vi "Assignment4_WashingMachine.vi"() -> ()   [LabVIEW 2024]
uses:
  WashingCycle.ctl
panel:
  in  "Mode":enum16{"Colourful", "Intensive", "Quick Wash"}(ring)
  in  "Start":bool
  out "Display":cluster{"Stage":string, "Time Remaining":dbl}
  in  "On/Off":bool
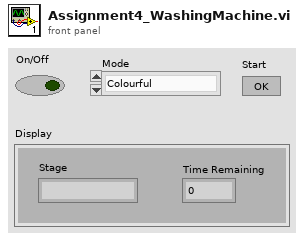
[diagram p1: front panel]
types:
  T1 = typedef "WashingCycle.ctl" = enum16{"Pre-rinse", "Main Washing", "Final Spin"}
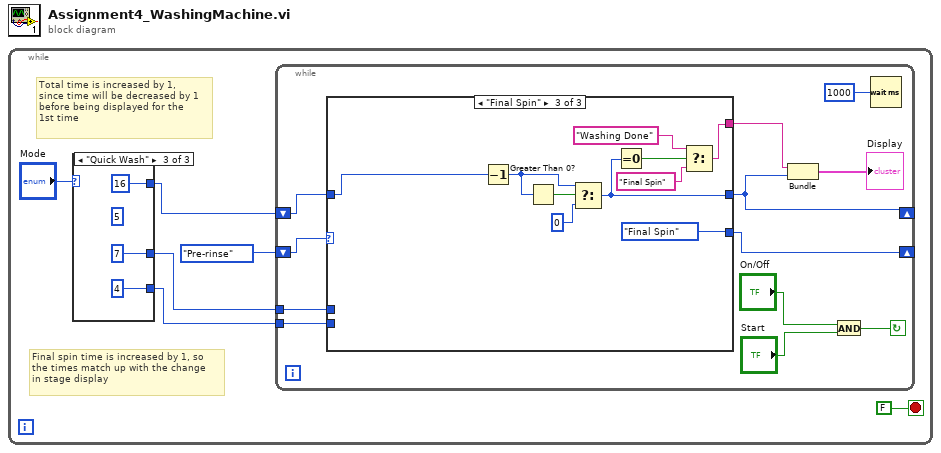
[diagram p0: block diagram]
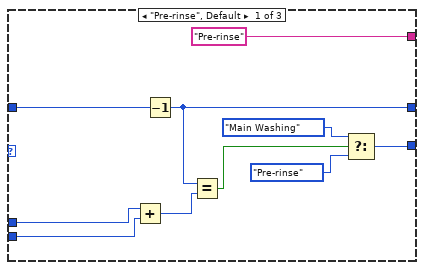
[diagram p2: hidden frame]
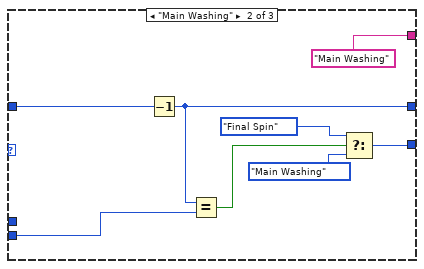
[diagram p3: hidden frame]
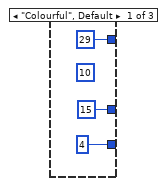
[diagram p4: hidden frame]
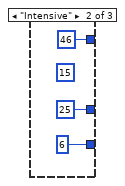
[diagram p5: hidden frame]
diagram:
  n1 = while {
    stop <- FALSE stop-if-true
    # "Final spin time is increased by 1, so\nthe times match up with the change\nin stage display"
    # "Total time is increased by 1,\nsince time will be decreased by 1\nbefore being displayed for the\n1st time"
    n2 = case shown="\"Quick Wash\"" "Mode" {
      tunnel: [15 25 7] -> w4
      tunnel: [4 6 4] -> w5
      tunnel: [29 46 16] -> w3
      frame "Colourful", Default {
        (unwired) 10
      }
      frame "Intensive" {
        (unwired) 15
      }
      frame "Quick Wash" {
        (unwired) 5
      }
    }
    n3 = while {
      shift-right: [w15] -> _
      shift-left: WashingCycle."Pre-rinse" -> [w16]
      tunnel: w5 -> [w14]
      tunnel: w4 -> [w13]
      shift-right: [w12] -> _
      shift-left: w3 -> [w11]
      stop <- w8 continue-if-true
      n4 = case shown="\"Final Spin\"" w16 {
        tunnel: [w25 w36 WashingCycle."Final Spin"] -> w15
        tunnel: ["Pre-rinse" "Main Washing" w45] -> w17
        tunnel: [w19 w29 w44] -> w12
        tunnel: w11 -> [w20 w30 w37]
        tunnel: w14 -> [w26 w34 _]
        tunnel: w13 -> [w27 _ _]
        frame "Pre-rinse", Default {
          n5 = Add(x=w27, y=w26) -> (x+y=w22:i32)
          n6 = Decrement(x=w20) -> (x-1=w19:i32)
          n7 = Equal?(x=w19, y=w22) -> (x = y?=w21:bool)
          n8 = Select(t=WashingCycle."Main Washing", s=w21, f=WashingCycle."Pre-rinse") -> (s? t:f=w25:T1)
        }
        frame "Main Washing" {
          n9 = Decrement(x=w30) -> (x-1=w29:i32)
          n10 = Equal?(x=w29, y=w34) -> (x = y?=w31:bool)
          n11 = Select(t=WashingCycle."Final Spin", s=w31, f=WashingCycle."Main Washing") -> (s? t:f=w36:T1)
        }
        frame "Final Spin" {
          n12 = Decrement(x=w37) -> (x-1=w38:i32)
          n13 = Greater Than 0?(x=w38) -> (x > 0?=w39:bool)
          n14 = Select(t=w38, s=w39, f=0) -> (s? t:f=w44:i32)
          n15 = Equal To 0?(x=w44) -> (x = 0?=w42:bool)
          n16 = Select(t="Washing Done", s=w42, f="Final Spin") -> (s? t:f=w45:string)
        }
      }
      n17 = Bundle(w17, w12) -> (→"Display":cluster{string, i32})  [unwired: 1 in]
      n18 = And(x="On/Off", y="Start") -> (x .and. y?=w8:bool)
      n19 = Wait (ms)(milliseconds to wait=u32 1000) -> ()  [unwired: 1 out]
    }
  }
